vi "Velocity_Profile.vi"(0 "Set Point":dbl(slide)=1510.204081632653 scale=-2000.0..2000.0, 1 "Rate Feedback":bool, 2 "Reset":bool, 3 "corr":bool, 5 "Position Sense":dbl(slide) scale=-2000.0..2000.0, 7 "Rate Sense":dbl(slide) scale=-1000.0..1000.0, 9 "coerce":dbl=1.0, 11 "Velocity Profile":dbl[][](array[numeric])=[[50.0, 75.0, 0.05], [100.0, 150.0, 0.1], [250.0, 400.0, 0.2], [500.0, inf, 0.2]]) -> (4 "Motor":dbl, 8 "arrived":bool, 15 "gear":i32)   [LabVIEW 2015]
doc: "VI DESCRIPTION:\n\nThis VI provides control of a motor speed via a 'velocity profile'. It requires a sensor input that is used to determine current position relative to a target position. VI output (Motor Out) will\nbe a function of how far the current distance is from the target, as prescribed by the input profile array. \n\nThe motor value can be profiled to be progressively reduced as the target distance \nis approached, like a P controller, but the motor value will not reduce to zero until the target is reached, ensuring the objective is reached.\n\nWhen position is near the hi or lo limit, the output can be no higher than a 'slow'\nvalue if (and only if) the position is continuing toward that limit - this reduces momentum prior to reaching a hard limit, which reduces positional overshoot. Output will become zero \nupon reaching a limit, but still allow for a reverse motor command to move position away from the limit.\n\nUse this only when the motor is NOT in a control loop (i.e. when under direct control from joystick). To limit motor travel when using a control loop, simply coerce the setpoint to limits."
panel:
  out "Accel":dbl
  out "Rate":dbl
  out "Waveform Chart":dbl(graph)
  # "Range"
  # "Rate"
  # "Accel"
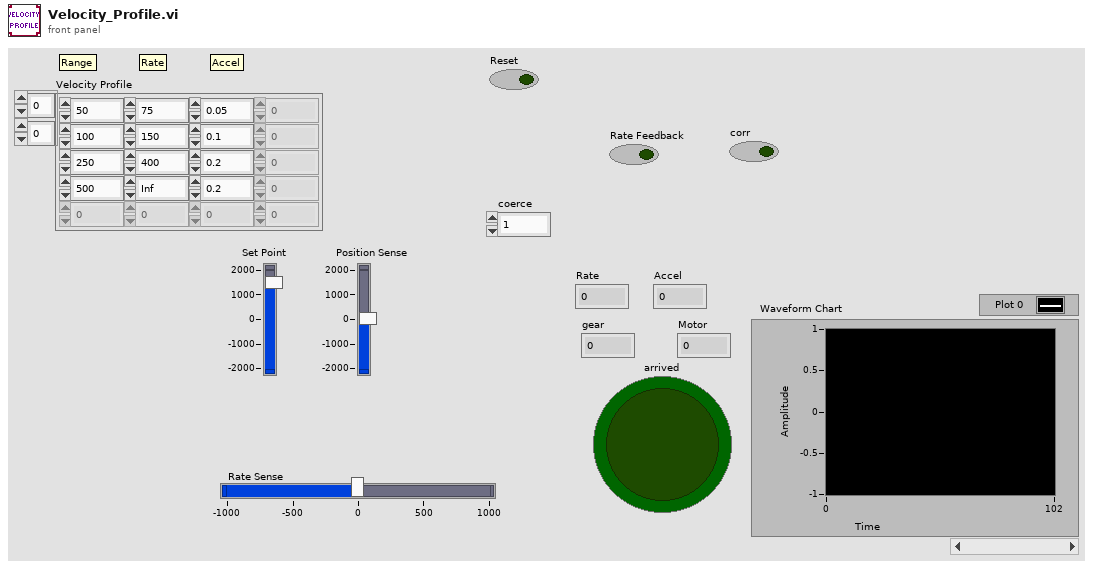
[diagram p1: front panel]
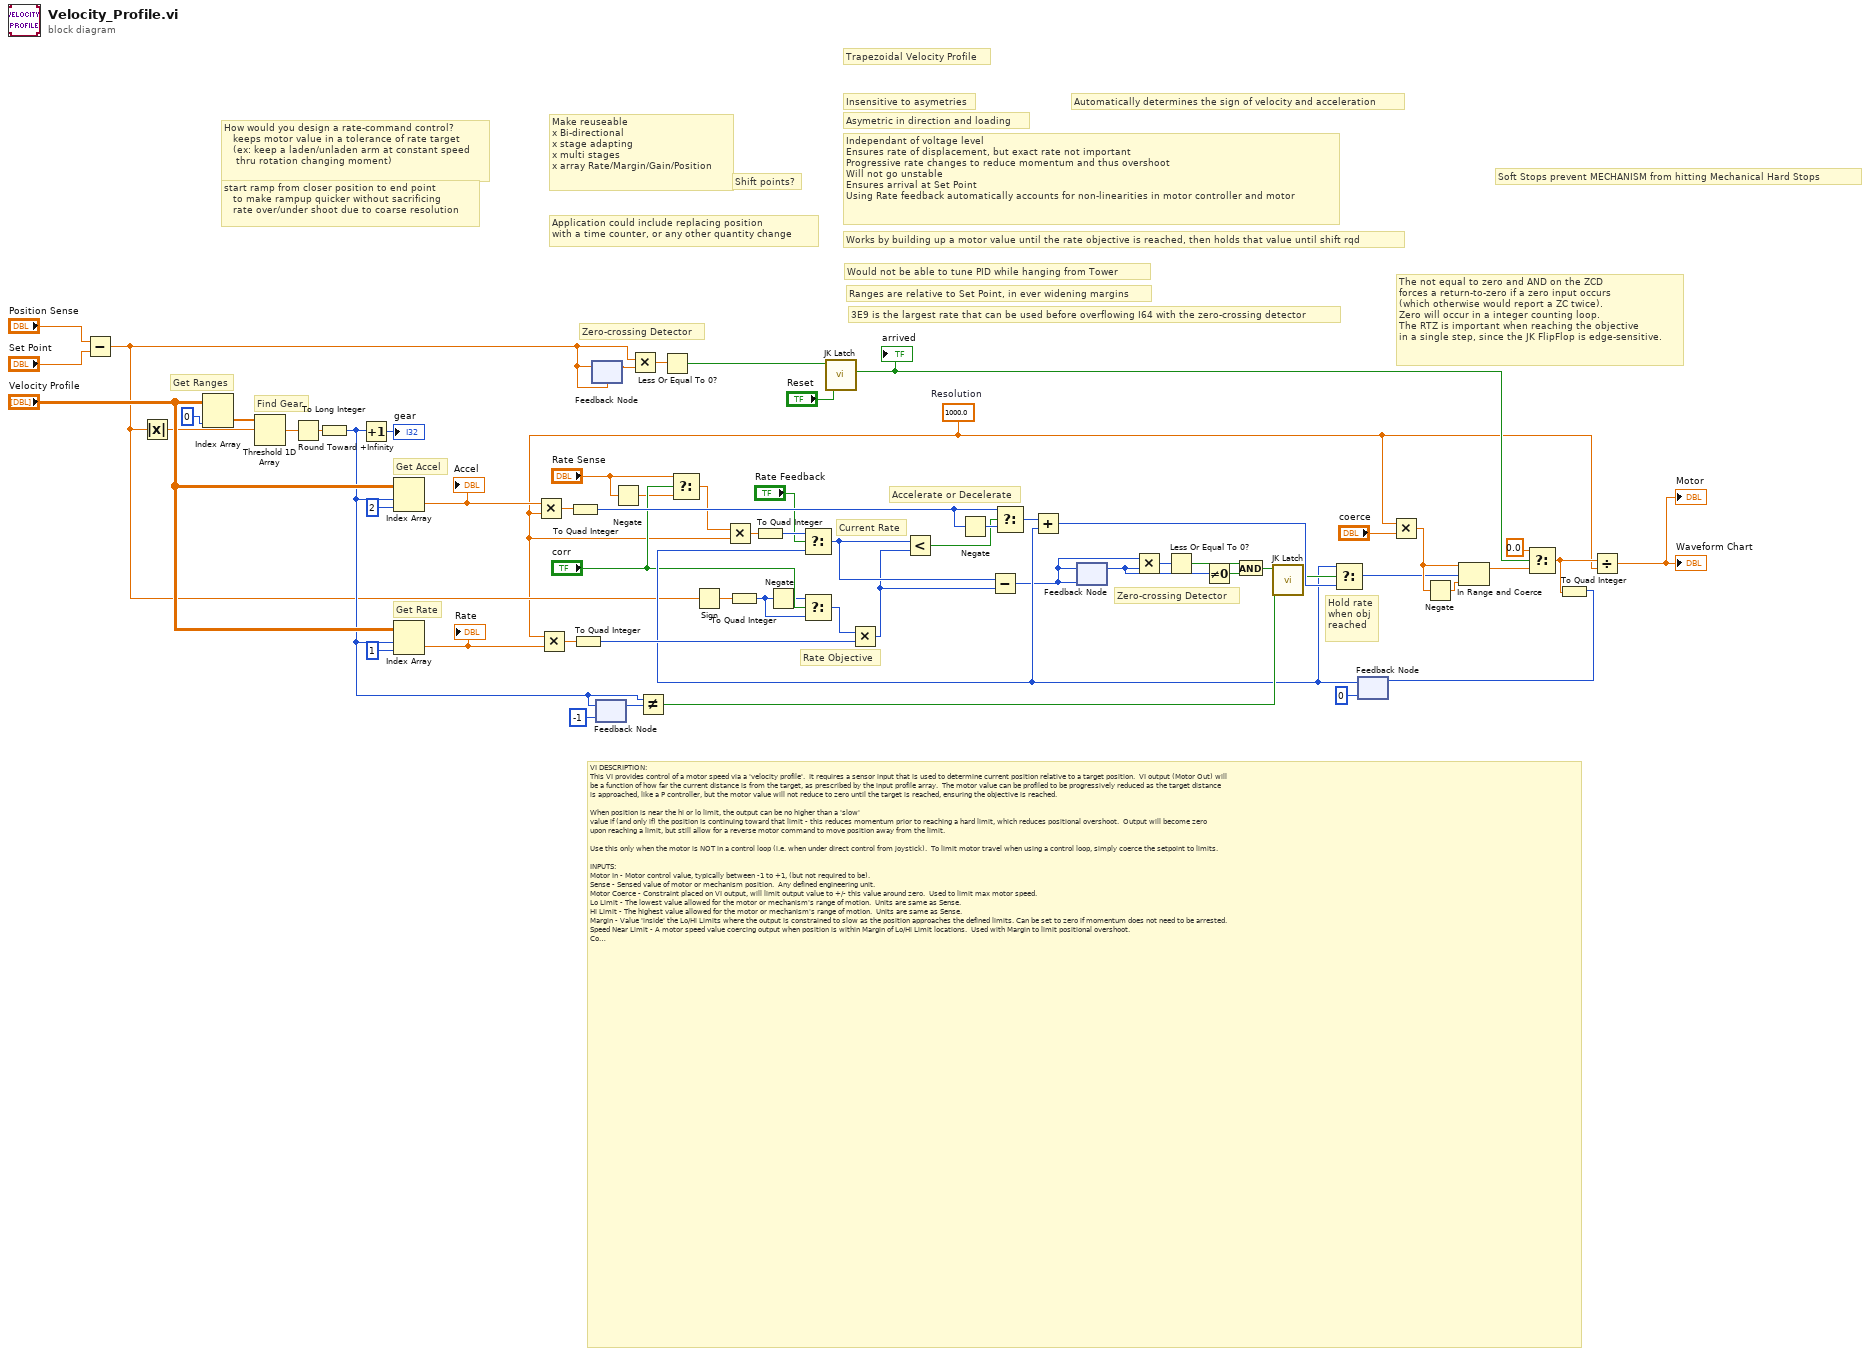
[diagram p0: block diagram]
diagram:
  w3 = 1000.0  # Resolution
  # "The not equal to zero and AND on the ZCD\nforces a return-to-zero if a zero input occurs\n(which otherwise would report a ZC twice).\nZero will occur in a integer counting loop.\nThe RTZ is important when reaching the objective\nin a single step, since the JK FlipFlop is edge-sensitive."
  # "Application could include replacing position\nwith a time counter, or any other quantity change"
  # "Hold rate\nwhen obj\nreached"
  # "Accelerate or Decelerate"
  # "Current Rate"
  # "Automatically determines the sign of velocity and acceleration"
  # "Zero-crossing Detector"
  # "Zero-crossing Detector"
  # "Rate Objective"
  # "3E9 is the largest rate that can be used before overflowing I64 with the zero-crossing detector"
  # "Ranges are relative to Set Point, in ever widening margins"
  # "Would not be able to tune PID while hanging from Tower"
  # "Get Accel"
  # "Get Rate"
  # "Find Gear"
  # "Get Ranges"
  # "Shift points?"
  # "How would you design a rate-command control?\n   keeps motor value in a tolerance of rate target\n   (ex: keep a laden/unladen arm at constant speed\n    thru rotation changing moment)"
  # "Trapezoidal Velocity Profile"
  # "Insensitive to asymetries"
  # "Works by building up a motor value until the rate objective is reached, then holds that value until shift rqd"
  # "start ramp from closer position to end point\n   to make rampup quicker without sacrificing\n   rate over/under shoot due to coarse resolution"
  # "Make reuseable\nx Bi-directional\nx stage adapting\nx multi stages\nx array Rate/Margin/Gain/Position"
  # "Independant of voltage level\nEnsures rate of displacement, but exact rate not important\nProgressive rate changes to reduce momentum and thus overshoot\nWill not go unstable\nEnsures arrival at Set Point\nUsing Rate feedback automatically accounts for non-linearities in motor controller and motor"
  # "Asymetric in direction and loading"
  # "VI DESCRIPTION:\nThis VI provides control of a motor speed via a 'velocity profile'.  It requires a sensor input that is used to determine current position relative to a target position.  VI output (Motor Out) will\nbe a function of how far the current distance is from the target, as prescribed by the input profile array.  The motor value can be profiled to be progressively reduced as the target distance \nis approached, like a P controller, but the motor value will not reduce to zero until the target is reached, ensuring the objective is reached.\n\nWhen position is near the hi or lo limit, the output can be no higher than a 'slow'\nvalue if (and only if) the position is continuing toward that limit - this reduces momentum prior to reaching a hard limit, which reduces positional overshoot.  Output will become zero \nupon reaching a limit, but still allow for a reverse motor command to move position away from the limit.\n\nUse this only when the motor is NOT in a control loop (i.e. when under direct control from joystick).  To limit motor travel when using a control loop, simply coerce the setpoint to limits.\n\nINPUTS:\nMotor In - Motor control value, typically between -1 to +1, (but not required to be).\nSense - Sensed value of motor or mechanism position.  Any defined engineering unit.\nMotor Coerce - Constraint placed on VI output, will limit output value to +/- this value around zero.  Used to limit max motor speed.\nLo Limit - The lowest value allowed for the motor or mechanism's range of motion.  Units are same as Sense.\nHi Limit - The highest value allowed for the motor or mechanism's range of motion.  Units are same as Sense.\nMargin - Value 'inside' the Lo/Hi Limits where the output is constrained to slow as the position approaches the defined limits. Can be set to zero if momentum does not need to be arrested.\nSpeed Near Limit - A motor speed value coercing output when position is within Margin of Lo/Hi Limit locations.  Used with Margin to limit positional overshoot.\nCorrelation - Set to True (default) for positive correlation between the signs of motor value and resultant sensor change.  Set to False if positive motor values cause decreasing sensor values.\nDisable Softstops - Set to True to over ride the softstop behavor and pass Motor In directly to Motor Out.\nDisable Motor - Set to True to send value zero to Motor Output.  If both Disables are selected, Disable Motor takes precedence over Disable Softstops.\n\nOUTPUTS:\nMotor Out - Motor control value modified by VI behavior.\nAt Lo - Boolean indicating status of sensed position, True if equal or lower than Lo Limit.\nAt Hi - Boolean indicating status of sensed position, True if equal or higher than Hi Limit.\n\nIMPLEMENTATION:\nDo not use in a control loop, instead use setpoint coercion for this situation.  For direct motor control:\nDetermine the correlation of the mechanical arrangement; if positive motor values cause increasing sensor values, set Correlation to True.\nDetermine the physical limits of the mechanism and set Lo and Hi Limits just short of these limits, by an amount that will accomodate any small overshoot that might remain after tuning.\nTo limit positional overshoot, create a region just inside each limit to slow the motor by setting Margin.\nSet Speed Near Limit to a value slow enough to bring the mechanism to a stop prior to reaching physical limits.\nSet Motor Coerce to the maximum speed that the mechanism is allowed to travel.\nExperimentally determine values that minimize the Margin region and maximize Speed Near Limit, without striking the mechanism's physical limits when approaching at full speed.\n\n\nFIRST Team 836, RoboBees"
  # "Soft Stops prevent MECHANISM from hitting Mechanical Hard Stops"
  n1 = Subtract(x="Position Sense", y="Set Point") -> (x-y=w7:dbl)
  n2 = Absolute Value(x=w7) -> (abs(x)=w46:dbl)
  n3 = Index Array(array="Velocity Profile", index (col)=0 ("disabled index (col)")) -> (element=w52:dbl[])  [unwired: 1 in]
  n4 = Threshold 1D Array(2:w46, 3:w52) -> (0:w53:dbl)  [unwired: 1 in]
  n5 = Round Toward +Infinity(x=w53) -> (ceil(x): smallest int >= x=w45:dbl)
  n6 = To Long Integer(number=w45) -> (32bit integer=w44:i32)
  n7 = Increment(x=w44) -> (x+1=→"gear":i32)
  n8 = Index Array(array="Velocity Profile", index (row)=w44, index (col)=2 ("disabled index (col)")) -> (element=w33:dbl)
  "Accel" <- w33
  n9 = Index Array(array="Velocity Profile", index (row)=w44, index (col)=1 ("disabled index (col)")) -> (element=w30:dbl)
  "Rate" <- w30
  n10 = Multiply(x=w33, y=w3) -> (x*y=w32:dbl)
  n11 = Multiply(x=w3, y=w30) -> (x*y=w31:dbl)
  n12 = To Quad Integer(1:w32) -> (0:w36:i64)
  n13 = To Quad Integer(1:w31) -> (0:w35:i64)
  n14 = feedback #1(w7) -> (w63:dbl)
  n15 = feedback-in #1(w7) -> ()
  n16 = feedback #2(-1) -> (w56:i32)
  n17 = feedback-in #2(w44) -> ()
  n18 = Negate(x="Rate Sense") -> (-x=w20:dbl)
  n19 = Multiply(x=w7, y=w63) -> (x*y=w62:dbl)
  n20 = Not Equal?(x=w44, y=w56) -> (x != y?=w39:bool)
  n21 = Less Or Equal To 0?(x=w62) -> (x <= 0?=w42:bool)
  n22 = Select(t="Rate Sense", s="corr", f=w20) -> (s? t:f=w9:dbl)
  n23 = Sign(1:w7) -> (0:w22:dbl)
  n24 = Multiply(x=w9, y=w3) -> (x*y=w10:dbl)
  n25 = To Quad Integer(1:w22) -> (0:w5:i64)
  n26 = To Quad Integer(1:w10) -> (0:w26:i64)
  n27 = Negate(x=w5) -> (-x=w6:i64)
  n28 = Select(t=w6, s="corr", f=w5) -> (s? t:f=w38:i64)
  n29 = call <userlib>:"JK Latch.vi"("Reset"="Reset", "Set"=w42) -> ("Q"=w41:bool)  [unwired: 5 in]
  "arrived" <- w41
  n30 = Multiply(x=w38, y=w35) -> (x*y=w11:i64)
  n31 = Negate(x=w36) -> (-x=w59:i64)
  n32 = feedback #3(i64 0) -> (w34:i64)
  n33 = Select(t=w26, s="Rate Feedback", f=w34) -> (s? t:f=w43:i64)
  n34 = Less?(x=w43, y=w11) -> (x < y?=w58:bool)
  n35 = Subtract(x=w43, y=w11) -> (x-y=w1:i64)
  n36 = Select(t=w36, s=w58, f=w59) -> (s? t:f=w13:i64)
  n37 = Add(x=w13, y=w34) -> (x+y=w57:i64)
  n38 = feedback #4(w1) -> (w2:i64)
  n39 = feedback-in #4(w1) -> ()
  n40 = Multiply(x=w1, y=w2) -> (x*y=w14:i64)
  n41 = Less Or Equal To 0?(x=w14) -> (x <= 0?=w16:bool)
  n42 = Not Equal To 0?(x=w2) -> (x != 0?=w17:bool)
  n43 = And(x=w16, y=w17) -> (x .and. y?=w15:bool)
  n44 = call <userlib>:"JK Latch.vi"("Reset"=w39, "Set"=w15) -> ("Q"=w55:bool)  [unwired: 5 in]
  n45 = Select(t=w34, s=w55, f=w57) -> (s? t:f=w25:i64)
  n46 = Multiply(x=w3, y="coerce") -> (x*y=w28:dbl)
  n47 = Negate(x=w28) -> (-x=w37:dbl)
  n48 = In Range and Coerce(upper limit=w28, x=w25, lower limit=w37) -> (coerced(x)=w24:dbl)  [unwired: 1 out]
  n49 = Select(t=0.0, s=w41, f=w24) -> (s? t:f=w29:dbl)
  n50 = To Quad Integer(1:w29) -> (0:w27:i64)
  n51 = feedback-in #3(w27) -> ()
  n52 = Divide(x=w29, y=w3) -> (x/y=→"Motor" →"Waveform Chart":dbl)
